vi "Sequence.BuildSetup.vi"(8 "error in (no error)":errorcluster, 10 "Sequence Channels":T1, 11 "Sequence":refnum<k24>) -> (0 "error out":errorcluster, 3 "Sequence out":refnum<k24>)   [LabVIEW 2015, in "Single Station Execution.lvlib"]
uses:
  Single Station Execution.lvlib
  NationalInstruments.VeriStand.RealTimeSequenceDefinitionApi
  Types/Compiled.SequenceChannels.ctl
  Types/Channel.Properties.ctl
  Main.Constants.vi
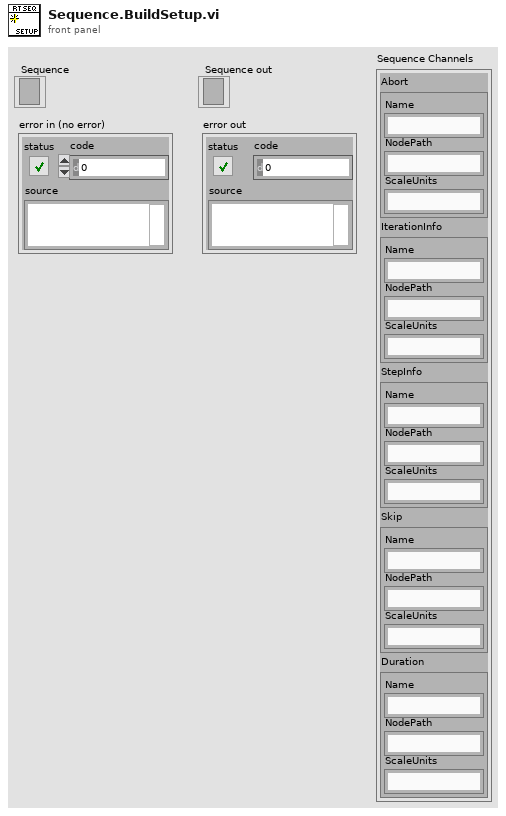
[diagram p1: front panel]
types:
  T1 = typedef "Single Station Execution.lvlib/Compiled.SequenceChannels.ctl" = cluster{"Abort":T2, "IterationInfo":T2, "StepInfo":T2, "Skip":T2, "Duration":T2}
  T2 = typedef "Single Station Execution.lvlib/Channel.Properties.ctl" = cluster{"Name":string, "NodePath":string, "ScaleUnits":string}
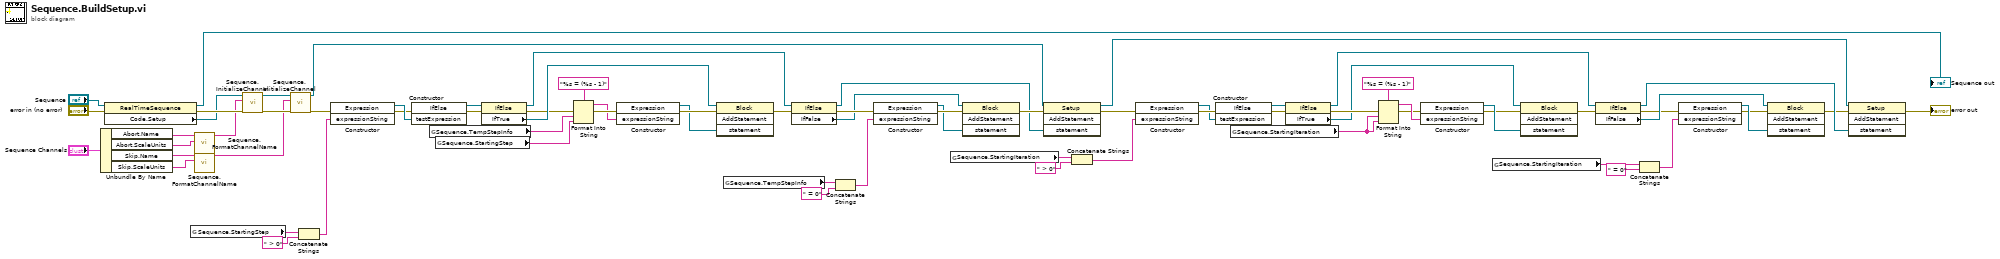
[diagram p0: block diagram]
diagram:
  n1 = Unbundle By Name("Sequence Channels") -> ("Abort.Name"=w10:string, "Abort.ScaleUnits"=w11:string, "Skip.Name"=w8:string, "Skip.ScaleUnits"=w7:string)
  n2 = property class="RealTimeSequence"(reference="Sequence", error in="error in (no error)") -> (reference out=→"Sequence out":refnum<k24>, error out=w13:errorcluster, "Code.Setup"=w12:refnum<k24>)
  n3 = global read "Main.Constants.vi" "Sequence.StartingStep"() -> (w66:string)
  n4 = call "Sequence.FormatChannelName.vi"("ScaleUnits"=w11, "Name"=w10) -> ("ChannelName"=w6:string)  [unwired: 9 in]
  n5 = call "Sequence.FormatChannelName.vi"("ScaleUnits"=w7, "Name"=w8) -> ("ChannelName"=w3:string)  [unwired: 9 in]
  n6 = call "Sequence.InitializeChannel.vi"("error in (no error)"=w13, "ChannelName"=w6, ".NET Refnum in"=w12) -> ("error out"=w5:errorcluster, ".NET Refnum out"=w4:refnum<k24>)  [unwired: 7 in]
  n7 = call "Sequence.InitializeChannel.vi"("error in (no error)"=w5, "ChannelName"=w3, ".NET Refnum in"=w4) -> ("error out"=w2:errorcluster, ".NET Refnum out"=w1:refnum<k24>)  [unwired: 7 in]
  n8 = Concatenate Strings(w66, " > 0" ("string")) -> (w64:string)
  n9 = constructor class="Expression"(error in=w2, "expressionString"=w64) -> (reference out=w68:refnum<k24>, error out=w67:errorcluster)  [unwired: 2 in, 2 out]
  n10 = constructor class="IfElse"(error in=w67, "testExpression"=w68) -> (reference out=w63:refnum<k24>, error out=w61:errorcluster)  [unwired: 2 in, 2 out]
  n11 = global read "Main.Constants.vi" "Sequence.TempStepInfo"() -> (w58:string)
  n12 = global read "Main.Constants.vi" "Sequence.StartingStep"() -> (w57:string)
  n13 = property class="IfElse"(reference=w63, error in=w61) -> (reference out=w52:refnum<k24>, error out=w59:errorcluster, "IfTrue"=w62:refnum<k24>)
  n14 = Format Into String(format string="%s = (%s - 1)", error in=w59, w58, w57) -> (resulting string=w54:string, error out=w56:errorcluster)  [unwired: 1 in]
  n15 = constructor class="Expression"(error in=w56, "expressionString"=w54) -> (reference out=w53:refnum<k24>, error out=w55:errorcluster)  [unwired: 2 in, 2 out]
  n16 = invoke class="Block" method="AddStatement"(reference=w62, error in=w55, "statement"=w53) -> (error out=w51:errorcluster)  [unwired: 1 in, 3 out]
  n17 = global read "Main.Constants.vi" "Sequence.TempStepInfo"() -> (w50:string)
  n18 = property class="IfElse"(reference=w52, error in=w51) -> (reference out=w42:refnum<k24>, error out=w46:errorcluster, "IfFalse"=w44:refnum<k24>)
  n19 = Concatenate Strings(w50, " = 0" ("expressionString")) -> (w47:string)
  n20 = constructor class="Expression"(error in=w46, "expressionString"=w47) -> (reference out=w45:refnum<k24>, error out=w48:errorcluster)  [unwired: 2 in, 2 out]
  n21 = global read "Main.Constants.vi" "Sequence.StartingIteration"() -> (w17:string)
  n22 = invoke class="Block" method="AddStatement"(reference=w44, error in=w48, "statement"=w45) -> (error out=w43:errorcluster)  [unwired: 1 in, 3 out]
  n23 = invoke class="Setup" method="AddStatement"(reference=w1, error in=w43, "statement"=w42) -> (reference out=w19:refnum<k24>, error out=w22:errorcluster)  [unwired: 1 in, 2 out]
  "error out" <- w22
  n24 = Concatenate Strings(w17, " > 0" ("string")) -> (w16:string)
  n25 = constructor class="Expression"(error in=w22, "expressionString"=w16) -> (reference out=w23:refnum<k24>, error out=w24:errorcluster)  [unwired: 2 in, 2 out]
  n26 = constructor class="IfElse"(error in=w24, "testExpression"=w23) -> (reference out=w25:refnum<k24>, error out=w26:errorcluster)  [unwired: 2 in, 2 out]
  n27 = global read "Main.Constants.vi" "Sequence.StartingIteration"() -> (w15:string)
  n28 = property class="IfElse"(reference=w25, error in=w26) -> (reference out=w20:refnum<k24>, error out=w28:errorcluster, "IfTrue"=w21:refnum<k24>)
  n29 = Format Into String(format string="%s = (%s - 1)", error in=w28, w15, w15) -> (resulting string=w31:string, error out=w29:errorcluster)  [unwired: 1 in]
  n30 = constructor class="Expression"(error in=w29, "expressionString"=w31) -> (reference out=w32:refnum<k24>, error out=w30:errorcluster)  [unwired: 2 in, 2 out]
  n31 = global read "Main.Constants.vi" "Sequence.StartingIteration"() -> (w14:string)
  n32 = invoke class="Block" method="AddStatement"(reference=w21, error in=w30, "statement"=w32) -> (error out=w33:errorcluster)  [unwired: 1 in, 3 out]
  n33 = property class="IfElse"(reference=w20, error in=w33) -> (reference out=w41:refnum<k24>, error out=w37:errorcluster, "IfFalse"=w39:refnum<k24>)
  n34 = Concatenate Strings(w14, " = 0" ("expressionString")) -> (w36:string)
  n35 = constructor class="Expression"(error in=w37, "expressionString"=w36) -> (reference out=w38:refnum<k24>, error out=w35:errorcluster)  [unwired: 2 in, 2 out]
  n36 = invoke class="Block" method="AddStatement"(reference=w39, error in=w35, "statement"=w38) -> (error out=w40:errorcluster)  [unwired: 1 in, 3 out]
  n37 = invoke class="Setup" method="AddStatement"(reference=w19, error in=w40, "statement"=w41) -> ()  [unwired: 1 in, 4 out]
